vi "状态告警区.vi"(11 "数组":u16[](array[numeric]) format="%04xH") -> (3 "状态告警区":T1)   [LabVIEW 2016, in "氨氮总磷.lvlib"]
panel:
  # "共占用29 WORD"
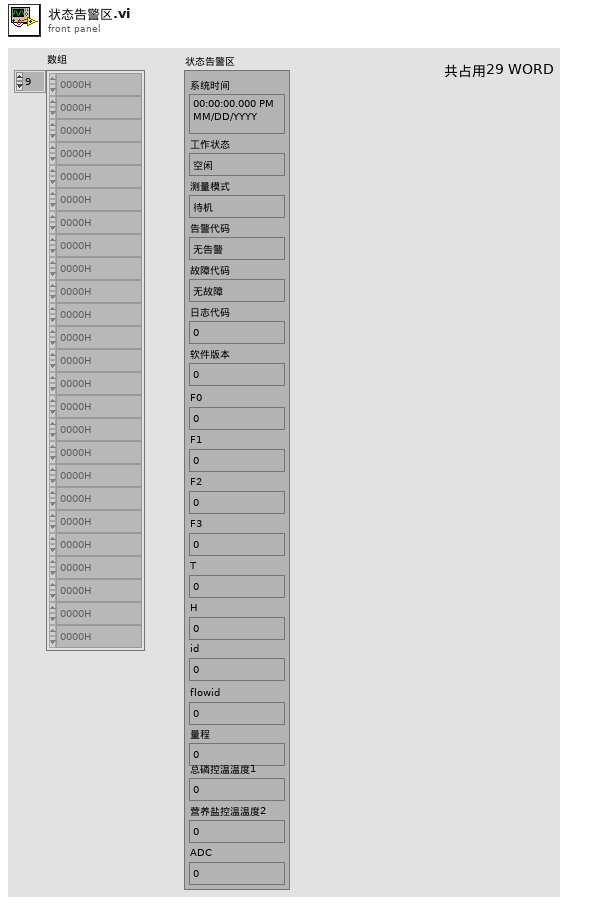
[diagram p1: front panel]
types:
  T1 = cluster{"系统时间":timestamp, "工作状态":enum16{"空闲", "水样测试", "标样核查", "零点核查", "跨度核查", "空白测试", "平行样测试", "加标回收", "空白校准", "标样校准", "初始化（清洗）"}, "测量模式":enum16{"待机", "连续模式", "周期模式", "定点模式", "受控模式", "手动模式"}, "告警代码":enum16{"无告警", "缺试剂告警", "缺水样告警", "缺蒸馏水告警", "缺标液告警", "仪表漏液告警", "标定异常告警", "超量程告警", "加热异常", "低试剂预警", "超上限告警", "超下限告警", "仪表内部其他异常", "滴定异常告警", "电极异常告警", "量程切换告警", "参数设置告警", "PH电极电位异常", "电导率电极异常", "浊度光度异常", "溶解氧电极异常", "溶解氧光强异常", "温度异常告警", "PH异常告警", "溶解氧异常告警", "电导率异常告警", "浊度异常告警", "叶绿素异常告警", "藻密度异常告警", "蓝绿藻异常告警", "ORP异常告警", "氨氮异常告警", "清洁刷异常告警", "SD卡异常告警", "蓝牙异常告警", "Wifi异常告警", "流程异常告警"}, "故障代码":enum16{"无故障", "电机故障", "温度故障", "通讯故障", "滴定故障"}, "日志代码":u16, "软件版本":u16, "F0":sgl, "F1":sgl, "F2":sgl, "F3":sgl, "T":sgl, "H":sgl, "id":u16, "flowid":u16, "量程":u16, "总磷控温温度1":sgl, "营养盐控温温度2":sgl, "ADC":sgl}
  T2 = cluster{"time stamp":timestamp, "WORD":u16, "WORD":u16, "WORD":u16, "WORD":u16, "WORD":u16, "WORD":u16, "FLOAT":sgl, "FLOAT":sgl, "FLOAT":sgl, "FLOAT":sgl, "FLOAT":sgl, "FLOAT":sgl, "WORD":u16, "WORD":u16, "WORD":u16, "FLOAT":sgl, "FLOAT":sgl, "WORD":u16}
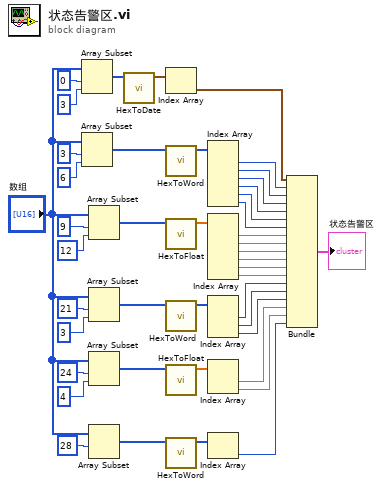
[diagram p0: block diagram]
diagram:
  n1 = Array Subset(array="数组", index=0 ("索引"), length=3 ("长度")) -> (w42:u16[])
  n2 = Array Subset(array="数组", index=3 ("索引"), length=6 ("长度")) -> (w37:u16[])
  n3 = Array Subset(array="数组", index=9 ("索引"), length=12 ("长度")) -> (w27:u16[])
  n4 = Array Subset(array="数组", index=21 ("索引"), length=3 ("索引")) -> (w17:u16[])
  n5 = Array Subset(array="数组", index=24 ("索引"), length=4 ("长度")) -> (w7:u16[])
  n6 = Array Subset(array="数组", index=28 ("索引")) -> (w5:u16[])  [unwired: 1 in]
  n7 = call "HexToDate.vi"("数组"=w42) -> ("DATE"=w39:timestamp[])  [unwired: 10 in]
  n8 = Index Array(array=w39) -> (element=w38:timestamp)  [unwired: 1 in]
  n9 = call "HexToWord.vi"("数组"=w37) -> ("WORD"=w36:u16[])  [unwired: 10 in]
  n10 = call "HexToFloat.vi"("数组"=w27) -> ("FLOAT"=w26:sgl[])  [unwired: 10 in]
  n11 = call "HexToWord.vi"("数组"=w17) -> ("WORD"=w16:u16[])  [unwired: 10 in]
  n12 = call "HexToFloat.vi"("数组"=w7) -> ("FLOAT"=w6:sgl[])  [unwired: 10 in]
  n13 = call "HexToWord.vi"("数组"=w5) -> ("WORD"=w4:u16[])  [unwired: 10 in]
  n14 = Index Array(array=w36) -> (element #1=w35:u16, element #2=w34:u16, element #3=w33:u16, element #4=w32:u16, element #5=w31:u16, element #6=w30:u16)  [unwired: 6 in]
  n15 = Index Array(array=w26) -> (element #1=w25:sgl, element #2=w24:sgl, element #3=w23:sgl, element #4=w22:sgl, element #5=w21:sgl, element #6=w20:sgl)  [unwired: 6 in]
  n16 = Index Array(array=w16) -> (element #1=w15:u16, element #2=w14:u16, element #3=w13:u16)  [unwired: 3 in]
  n17 = Index Array(array=w6) -> (element #1=w3:sgl, element #2=w2:sgl)  [unwired: 2 in]
  n18 = Index Array(array=w4) -> (element=w1:u16)  [unwired: 1 in]
  n19 = Bundle("time stamp"=w38, "WORD"=w35, "WORD"=w34, "WORD"=w33, "WORD"=w32, "WORD"=w31, "WORD"=w30, "FLOAT"=w25, "FLOAT"=w24, "FLOAT"=w23, "FLOAT"=w22, "FLOAT"=w21, "FLOAT"=w20, "WORD"=w15, "WORD"=w14, "WORD"=w13, "FLOAT"=w3, "FLOAT"=w2, "WORD"=w1) -> (→"状态告警区":T2)  [unwired: 1 in]
